vi "Front_to_access_test2.vi"() -> ()   [LabVIEW 2017]
uses:
  3d2c738f-2ce4-42c3-92bd-9b70d865882f.vi
panel:
  out "value out":errorcluster
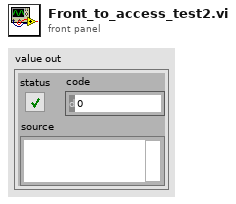
[diagram p1: front panel]
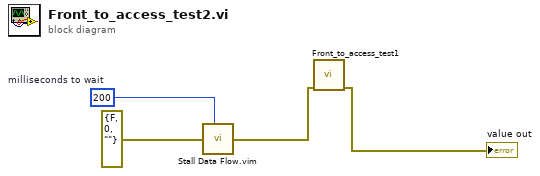
[diagram p0: block diagram]
diagram:
  w3 = u32 200  # milliseconds to wait
  n1 = call "Stall Data Flow.vim"("value in"=errorcluster {"status"=FALSE, "code"=0, "source"=""} ("error in (no error)"), "milliseconds to wait"=w3) -> ("value out"=w2:errorcluster)  [unwired: 1 out]
  n2 = call "Front_to_access_test1.vi"("error in (no error) 2"=w2) -> ("error in (no error)"=→"value out":errorcluster)  [unwired: 10 in]
